vi "Flatten Value.vi"(8 "Error In":errorcluster, 11 "String In":refnum<class "String.lvclass">) -> (0 "Error Out":errorcluster, 1 "Value":string, 3 "String Out":refnum<class "String.lvclass">)   [LabVIEW 2020, in "NI_VIAnCFGDataStructure.lvlib" / "String.lvclass"]
uses:
  <vilib>/addons/analyzer/VIAnCFGDataStructure/Data Types/String/String.lvclass
  <vilib>/addons/analyzer/VIAnCFGDataStructure/Data Types/String/String.lvclass/String.ctl
  <vilib>/addons/analyzer/VIAnCFGDataStructure/Tree Manager/API/Generate Hash.vi
  <vilib>/addons/analyzer/VIAnCFGDataStructure/Tree Manager/Tree.lvclass
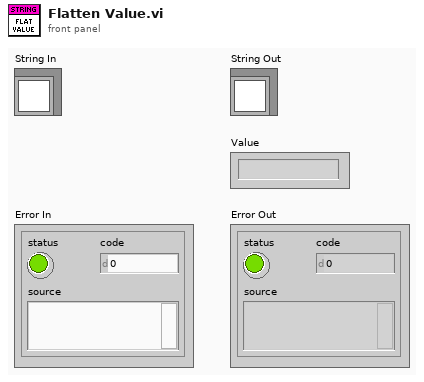
[diagram p1: front panel]
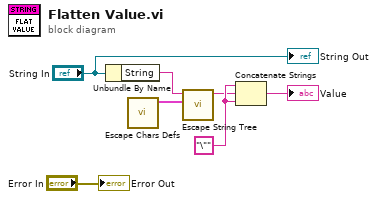
[diagram p0: block diagram]
diagram:
  w5 = "\"" ("string")
  n1 = Unbundle By Name("String In") -> ("String"=w2:string)
  n2 = call <vilib>:"Escape Chars Defs.vi"() -> ("Escapes"=w3:cluster{"String":string, "Escape":string}[])  [unwired: 11 in]
  n3 = call <vilib>:"Escape String Tree.vi"("Escapes"=w3, "String In"=w2) -> ("String Out"=w1:string)  [unwired: 9 in]
  n4 = Concatenate Strings(w5, w1, w5) -> (→"Value":string)
  "String Out" <- "String In"
  "Error Out" <- "Error In"
